vi "Calculate Temp Sensing.vi"() -> ()   [LabVIEW 2013]
uses:
  <vilib>/Analysis/NI_AALBase.lvlib
panel:
  in  "Numeric":i32
  out "Array":dbl[](array[numeric])
  out "variance":dbl format="%0.2f"
  out "standard deviation":dbl format="%0.2f"
  out "mean":dbl format="%0.2f"
  in  "array":dbl[][](array[numeric])=[[121.0, 193.0, 297.0, 391.0, 507.0, 612.0, 719.0, 857.0, 984.0], [120.0, 198.0, 294.0, 390.0, 505.0, 610.0, 727.0, 860.0, 987.0], [118.0, 199.0, 293.0, 390.0, 504.0, 612.0, 728.0, 861.0, 989.0], [119.0, 196.0, 295.0, 390.0, 506.0, 612.0, 729.0, 860.0, 990.0], [119.0, 196.0, 299.0, 393.0, 505.0, 612.0, 730.0, 860.0, 990.0], [118.0, 199.0, 298.0, 390.0, 505.0, 615.0, 728.0, 860.0, 988.0], [118.0, 198.0, 298.0, 393.0, 506.0, 616.0, 730.0, 862.0, 988.0], [118.0, 199.0, 297.0, 392.0, 508.0, 614.0, 730.0, 864.0, 986.0], [118.0, 197.0, 295.0, 393.0, 507.0, 613.0, 730.0, 864.0, 986.0], [119.0, 196.0, 296.0, 391.0, 506.0, 611.0, 730.0, 864.0, 986.0], [119.0, 197.0, 296.0, 392.0, 506.0, 616.0, 731.0, 865.0, 985.0], [117.0, 197.0, 297.0, 391.0, 505.0, 615.0, 732.0, 865.0, 983.0], [117.0, 198.0, 297.0, 391.0, 503.0, 616.0, 731.0, 865.0, 984.0], [118.0, 198.0, 297.0, 392.0, 504.0, 618.0, 730.0, 864.0, 984.0], [120.0, 200.0, 294.0, 392.0, 505.0, 618.0, 731.0, 865.0, 983.0], [118.0, 196.0, 294.0, 396.0, 507.0, 617.0, 731.0, 865.0, 983.0], [120.0, 198.0, 298.0, 394.0, 506.0, 616.0, 731.0, 867.0, 983.0], [121.0, 195.0, 297.0, 392.0, 504.0, 613.0, 732.0, 866.0, 979.0], [120.0, 196.0, 295.0, 390.0, 504.0, 610.0, 729.0, 867.0, 978.0], [122.0, 196.0, 297.0, 393.0, 504.0, 614.0, 732.0, 866.0, 981.0], [120.0, 199.0, 299.0, 393.0, 506.0, 614.0, 731.0, 866.0, 984.0], [120.0, 197.0, 298.0, 393.0, 506.0, 615.0, 730.0, 866.0, 984.0], [120.0, 197.0, 297.0, 391.0, 507.0, 616.0, 729.0, 867.0, 985.0], [120.0, 195.0, 298.0, 394.0, 508.0, 614.0, 726.0, 867.0, 986.0], [118.0, 197.0, 296.0, 393.0, 506.0, 611.0, 728.0, 868.0, 987.0], [118.0, 197.0, 297.0, 394.0, 506.0, 612.0, 726.0, 868.0, 986.0], [119.0, 197.0, 296.0, 397.0, 506.0, 614.0, 727.0, 864.0, 989.0], [120.0, 199.0, 296.0, 394.0, 510.0, 616.0, 727.0, 860.0, 986.0], [121.0, 198.0, 297.0, 396.0, 511.0, 615.0, 729.0, 858.0, 986.0], [118.0, 197.0, 297.0, 396.0, 508.0, 614.0, 727.0, 854.0, 989.0], [120.0, 197.0, 296.0, 396.0, 511.0, 616.0, 726.0, 853.0, 989.0], [121.0, 197.0, 298.0, 397.0, 510.0, 616.0, 726.0, 853.0, 989.0], [116.0, 198.0, 298.0, 397.0, 507.0, 617.0, 727.0, 854.0, 990.0], [123.0, 198.0, 296.0, 398.0, 509.0, 612.0, 730.0, 855.0, 990.0], [116.0, 197.0, 297.0, 395.0, 508.0, 611.0, 729.0, 857.0, 988.0], [121.0, 197.0, 297.0, 395.0, 509.0, 610.0, 728.0, 856.0, 986.0], [122.0, 199.0, 299.0, 396.0, 510.0, 613.0, 730.0, 856.0, 986.0], [119.0, 198.0, 298.0, 395.0, 510.0, 612.0, 728.0, 851.0, 986.0], [119.0, 196.0, 295.0, 396.0, 511.0, 613.0, 728.0, 852.0, 988.0], [121.0, 197.0, 295.0, 397.0, 511.0, 615.0, 725.0, 852.0, 988.0], [119.0, 193.0, 292.0, 396.0, 512.0, 613.0, 726.0, 852.0, 993.0], [119.0, 196.0, 296.0, 398.0, 513.0, 611.0, 726.0, 853.0, 989.0], [120.0, 197.0, 292.0, 398.0, 510.0, 613.0, 727.0, 855.0, 991.0], [119.0, 196.0, 294.0, 397.0, 512.0, 613.0, 727.0, 852.0, 993.0], [119.0, 197.0, 292.0, 399.0, 513.0, 612.0, 729.0, 852.0, 993.0], [121.0, 200.0, 294.0, 399.0, 510.0, 611.0, 729.0, 858.0, 993.0], [120.0, 199.0, 294.0, 399.0, 507.0, 609.0, 728.0, 855.0, 992.0], [119.0, 197.0, 295.0, 399.0, 510.0, 610.0, 729.0, 857.0, 994.0], [119.0, 196.0, 293.0, 400.0, 511.0, 610.0, 728.0, 857.0, 994.0], [117.0, 199.0, 295.0, 397.0, 511.0, 610.0, 729.0, 859.0, 993.0], [119.0, 198.0, 296.0, 400.0, 510.0, 611.0, 727.0, 858.0, 994.0], [119.0, 198.0, 293.0, 398.0, 511.0, 609.0, 727.0, 860.0, 992.0]]
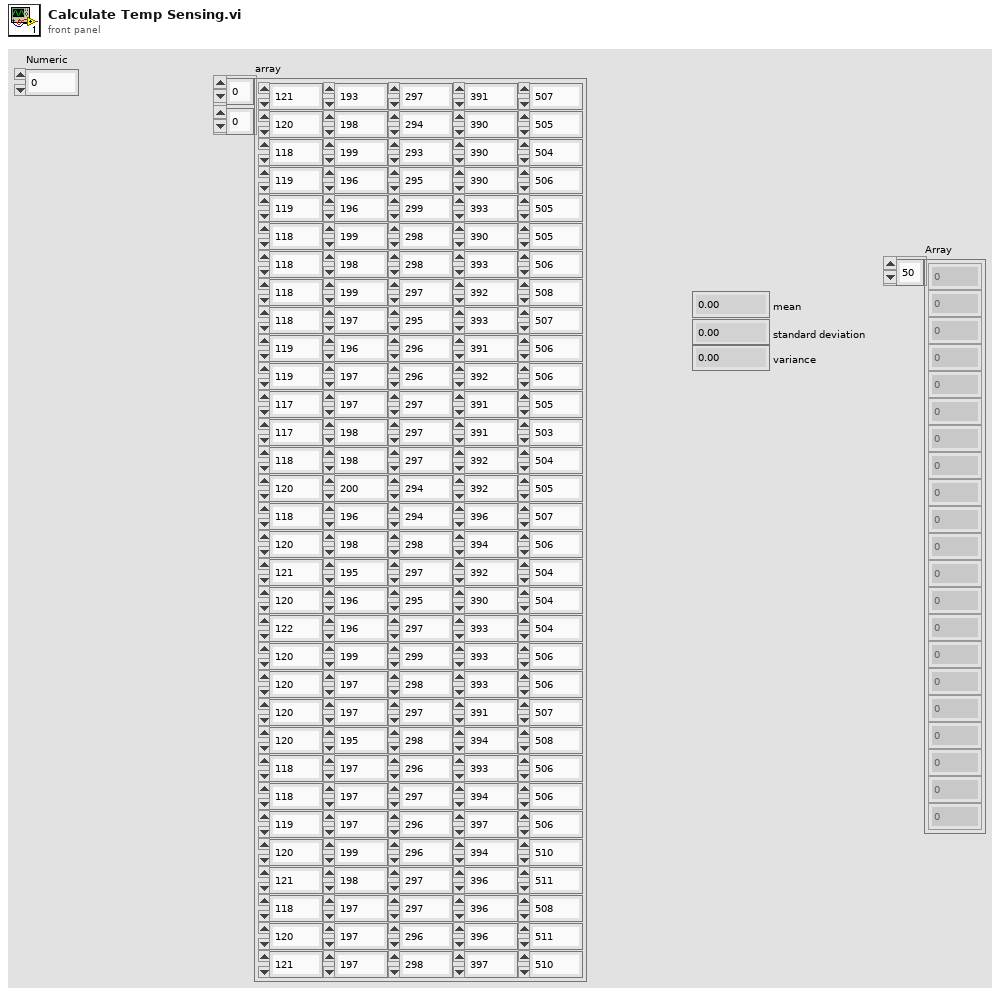
[diagram p1: front panel]
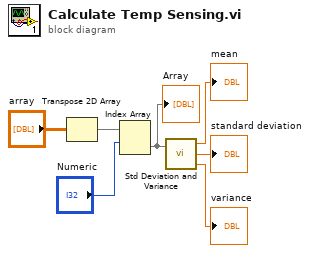
[diagram p0: block diagram]
diagram:
  n1 = Transpose 2D Array(2D array="array") -> (transposed array=w3:dbl[][])
  n2 = Index Array(array=w3, index (row)="Numeric") -> (element=w1:dbl[])  [unwired: 1 in]
  "Array" <- w1
  n3 = call <vilib>:"Std Deviation and Variance.vi"("X"=w1) -> ("mean"=→"mean":dbl, "standard deviation"=→"standard deviation":dbl, "variance"=→"variance":dbl)  [unwired: 1 in]
